vi "Autonomous.vi"() -> ()   [LabVIEW 2016]
doc: "This VI starts when autonomous period begins, and will automatically be terminated when it ends. You can carry out timed or sensor driven operations directly to I/O or to subsystems without needing to return to the caller."
uses:
  <vilib>/Rock Robotics/WPI/ThirdParty/CanMotor/TalonSRX/WPI_CANTalonSRX_BrakeOverride.ctl
  <vilib>/Rock Robotics/WPI/Utilities/WPI_GetSetVariantRefNum.vi
  <vilib>/Rock Robotics/Network Tables/NT Read String.vi
  <vilib>/Rock Robotics/Network Tables/NT Read Number.vi
  Winch/Implementation/Winch Globals.vi
  <vilib>/Rock Robotics/Network Tables/NT Read Boolean.vi
panel:
  in  "stop 3":bool
  in  "stop 2":bool
  out "x-y":u32
  in  "stop":bool
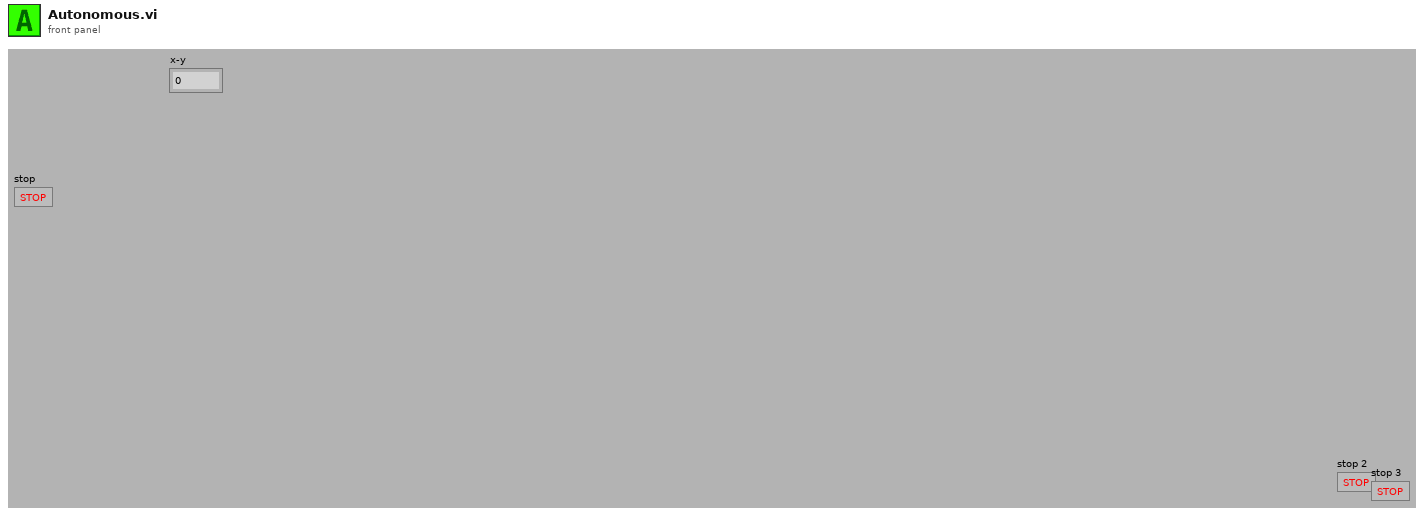
[diagram p1: front panel]
types:
  T1 = typedef "WPI_JoystickDevRef.ctl" = cluster{"Device":T2}
  T2 = typedef "WPI_JoystickDeviceEnum.ctl" = enum16{"USB 0", "USB 1", "USB 2", "USB 3", "USB 4", "USB 5"}
  T3 = typedef "WPI_CANTalonSRX_BrakeOverride.ctl" = enum8{"No Override", "Override to Coast", "Override to Brake"}
  T4 = typedef "WPI_RobotDriveDevRef.ctl" = cluster{"DevStatus":errorcluster, "Motors[]":T5[], "Square Inputs":bool, "Max Output":dbl}
  T5 = typedef "WPI_MotorControlDeviceRef.ctl" = cluster{"DeviceStatus":errorcluster, "Type":T6, "PWM":cluster{"PWM Channel":T7, "DeadBand":T8}, "CAN":cluster{"Device Number":u8, "SetOutput VI Ref":variant, "GetOutput VI Ref":variant, "Enable VI Ref":variant, "Disable VI Ref":variant, "Data":variant}, "Invert":bool}
  T6 = typedef "WPI_MotorControlType.ctl" = enum16{"PWM", "CAN"}
  T7 = typedef "FPGA_DIOPWMChannel.ctl" = enum8{"PWM 0", "PWM 1", "PWM 2", "PWM 3", "PWM 4", "PWM 5", "PWM 6", "PWM 7", "PWM 8", "PWM 9", "PWM MXP 0", "PWM MXP 1", "PWM MXP 2", "PWM MXP 3", "PWM MXP 4", "PWM MXP 5", "PWM MXP 6", "PWM MXP 7", "PWM MXP 8", "PWM MXP 9", "Invalid"}
  T8 = typedef "WPI_PWMDeadband.ctl" = cluster{"Name":string, "maxPositivePwm":i32, "minPositivePwm":i32, "centerPwm":i32, "maxNegativePwm":i32, "minNegativePwm":i32, "angularRange":u16}
  T9 = typedef "WPI_ServoDeviceRef.ctl" = cluster{"DeviceStatus":errorcluster, "PWM Channel":T7, "DeadBand":T8}
  T10 = typedef "Command Status Info.ctl" = cluster{"Name":string, "Status":T11, "notifier out":T12}
  T11 = typedef "Completion Status.ctl" = enum16{"Successful", "Aborted", "Incomplete"}
  T12 = typedef "Completion Notifier.ctl" = refnum<notifier>
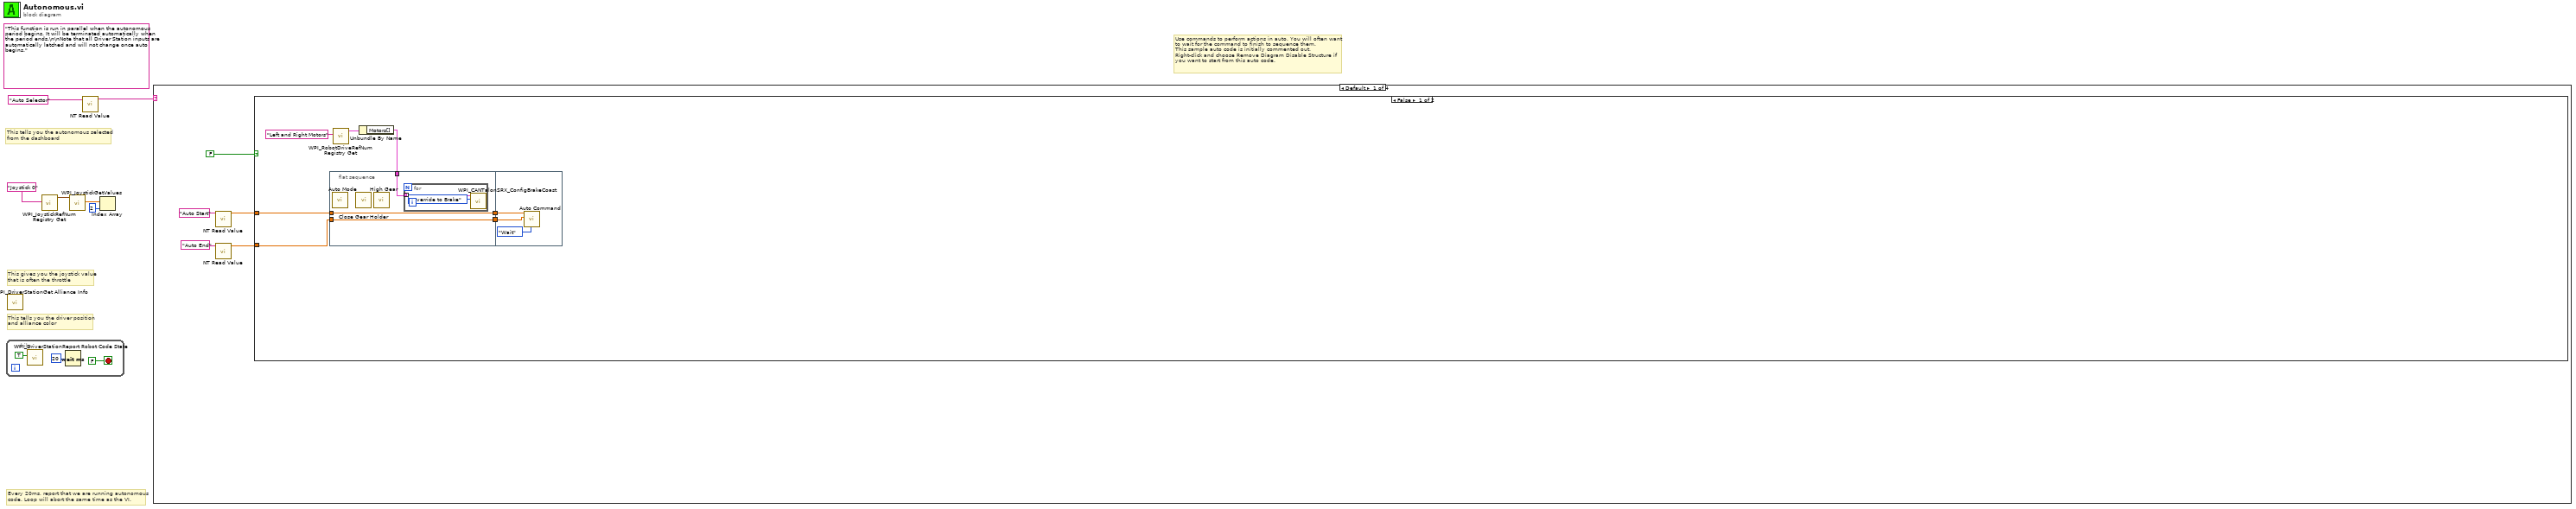
[diagram p0: block diagram]
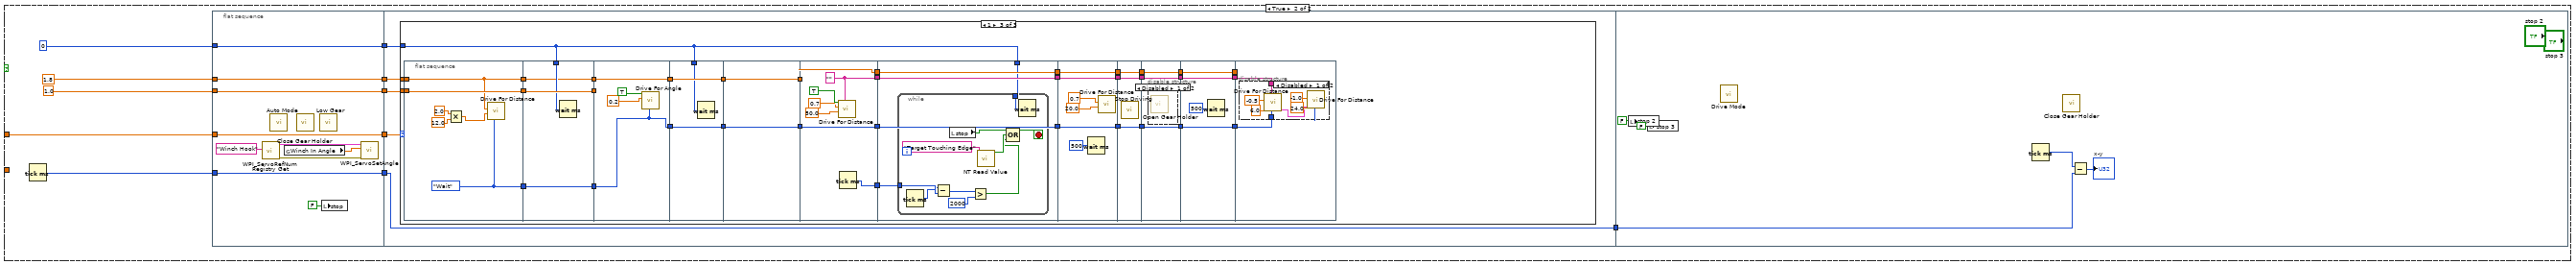
[diagram p2: hidden frame]
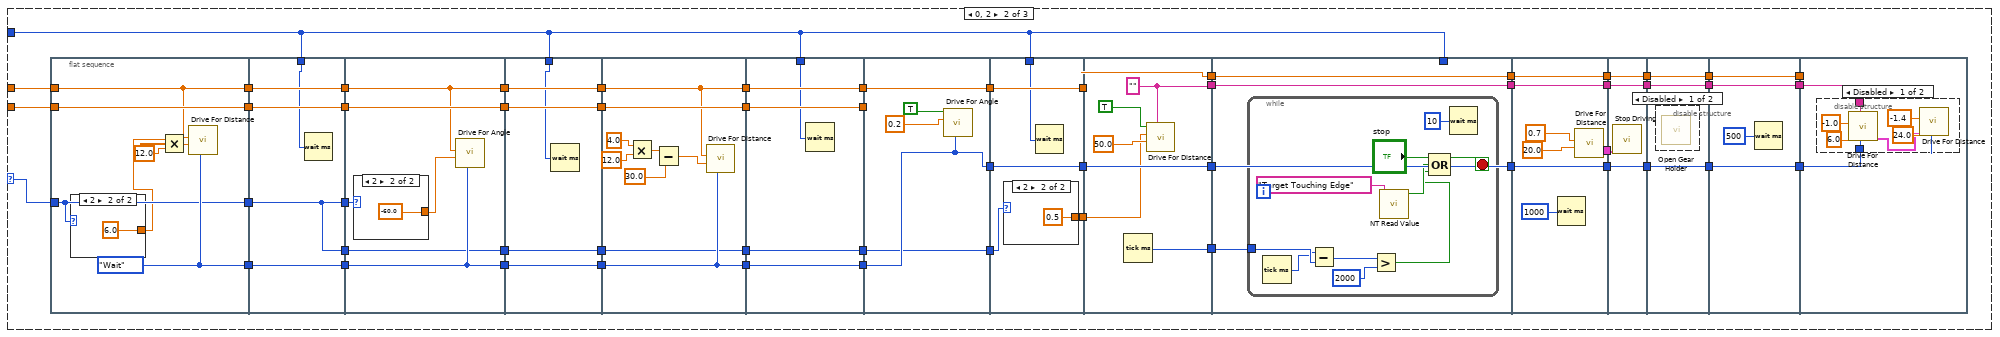
[diagram p4: hidden frame]
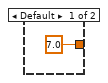
[diagram p5: hidden frame]
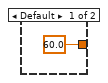
[diagram p6: hidden frame]
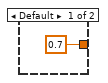
[diagram p7: hidden frame]
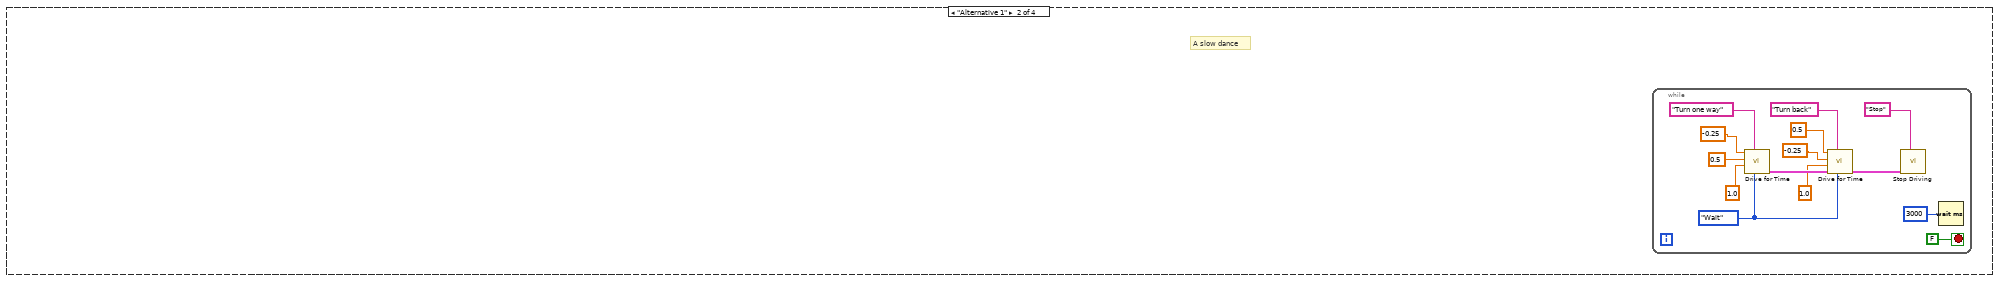
[diagram p12: hidden frame]
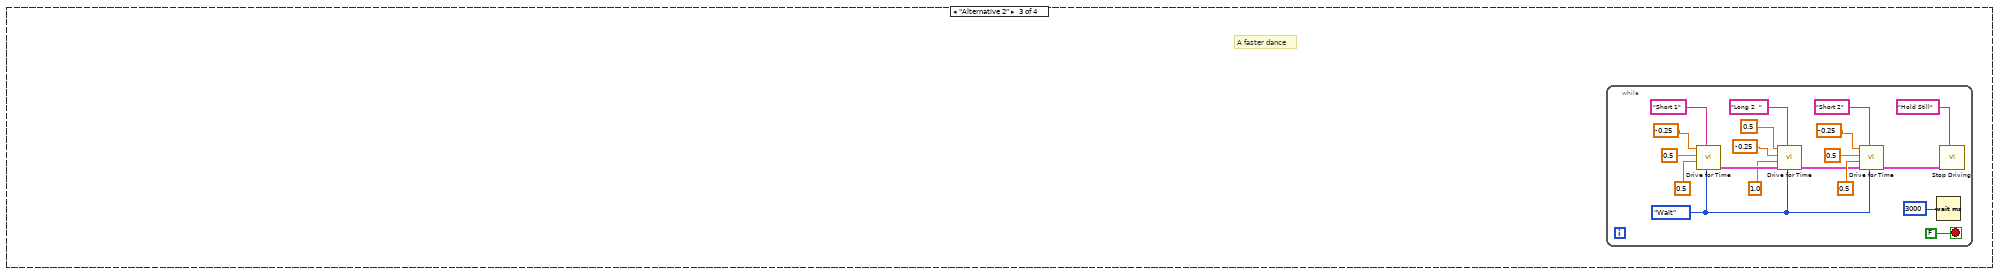
[diagram p13: hidden frame]
diagram:
  (unwired) "This function is run in parallel when the autonomous period begins. It will be terminated automatically when the period ends.\n\nNote that all Driver Station inputs are automatically latched and will not change once auto begins."
  # "This tells you the autonomous selected\nfrom the dashboard"
  # "Every 20ms, report that we are running autonomous\ncode. Loop will abort the same time as the VI."
  # "This gives you the joystick value\nthat is often the throttle"
  # "Use commands to perform actions in auto. You will often want\nto wait for the command to finish to sequence them.\nThis sample auto code is initially commented out. \nRight-click and choose Remove Diagram Disable Structure if\nyou want to start from this auto code."
  # "This tells you the driver position\nand alliance color"
  n1 = while {
    stop <- FALSE stop-if-true
    n2 = call <vilib>:"WPI_DriverStationReport Robot Code State.vi"("Autonomous"=TRUE) -> ()  [unwired: 10 in, 1 out]
    n3 = Wait (ms)(milliseconds to wait=u32 20) -> ()  [unwired: 1 out]
  }
  n4 = call <vilib>:"WPI_DriverStationGet Alliance Info.vi"() -> ()  [unwired: 12 out]
  n5 = call <vilib>:"WPI_JoystickRefNum Registry Get.vi"("refnum name"="Joystick 0") -> ("JoystickDevRef"=w5:T1)  [unwired: 1 in, 9 out]
  n6 = call <vilib>:"WPI_JoystickGetValues.vi"("JoystickDevRef"=w5) -> ("Axes"=w4:dbl[])  [unwired: 6 in, 4 out]
  n7 = call-poly <vilib>:"NT Read Value.vi"("Name"="Auto Selector") -> ("String"=w1:string)  [unwired: 9 in, 1 out]
  n8 = Index Array(array=w4, index=2) -> ()  [unwired: 1 out]
  n9 = case shown="Default" w1 {
    frame Default {
      n10 = call-poly <vilib>:"NT Read Value.vi"("Name"="Auto Start") -> ("Numeric"=w12:dbl)  [unwired: 9 in, 1 out]
      n11 = call-poly <vilib>:"NT Read Value.vi"("Name"="Auto End") -> ("Numeric"=w10:dbl)  [unwired: 9 in, 1 out]
      n12 = case shown="False" FALSE {
        tunnel: w12 -> [w21 w30]
        tunnel: w10 -> [w18 _]
        frame False {
          n13 = flat-sequence {
            tunnel: w21 -> [w24]
            tunnel: [w24] -> w20
            tunnel: w18 -> [w23]
            tunnel: [w23] -> w19
            tunnel: w15 -> [w22]
            tunnel: w20 -> [w29]
            tunnel: w19 -> [w27]
            frame #0 {
              n14 = call "Auto Mode.vi"() -> ()  [unwired: 12 in]
              n15 = call "Close Gear Holder.vi"() -> ()  [unwired: 12 in]
              n16 = call "High Gear.vi"() -> ()  [unwired: 12 in]
              n17 = for {
                tunnel: w22 -> [w25] mode=indexing
                n18 = call <vilib>:"WPI_CANTalonSRX_ConfigBrakeCoast.vi"("Brake / Coast Mode"=WPI_CANTalonSRX_BrakeOverride."Override to Brake", "CAN Talon SRX Ref"=w25) -> ()  [unwired: 8 in, 2 out]
              }
            }
            frame #1 {
              n19 = call "Auto Command.vi"("Synchronization"=enum16{"Start", "Wait"}."Wait", "End Position"=w27, "Start Position"=w29) -> ()  [unwired: 7 in, 2 out]
            }
          }
          n20 = call <vilib>:"WPI_RobotDriveRefNum Registry Get.vi"("refnum name"="Left and Right Motors") -> ("RobotDriveDevRef"=w16:T4)  [unwired: 9 in, 1 out]
          n21 = Unbundle By Name(w16) -> ("Motors[]"=w15:T5[])
        }
        frame True {
          n22 = Tick Count (ms)() -> (millisecond timer value=w31:u32)
          n23 = flat-sequence {
            tunnel: w31 -> [w47]
            tunnel: u32 0 ("milliseconds to wait") -> [w48]
            tunnel: 1.0 ("Speed") -> [w49]
            tunnel: 1.8 ("Speed") -> [w50]
            tunnel: [w50] -> w40
            tunnel: [w49] -> w39
            tunnel: [w48] -> w38
            tunnel: [w47] -> w37
            tunnel: [w42] -> w36
            tunnel: w30 -> [w42]
            tunnel: w40 -> [w55]
            tunnel: w39 -> [w54]
            tunnel: w38 -> [w53]
            tunnel: w37 -> [w52]
            tunnel: [w52] -> w35
            tunnel: w36 -> [w51]
            tunnel: w35 -> [w314]
            frame #0 {
              n24 = call <vilib>:"WPI_ServoRefNum Registry Get.vi"("refnum name"="Winch Hook") -> ("error out"=w46:errorcluster, "ServoDeviceRef"=w45:T9)  [unwired: 9 in]
              n25 = call "Auto Mode.vi"() -> ()  [unwired: 12 in]
              n26 = global read "Winch Globals.vi" "Winch In Angle"() -> (w43:dbl)
              n27 = call "Close Gear Holder.vi"() -> ()  [unwired: 12 in]
              n28 = call "Low Gear.vi"() -> ()  [unwired: 12 in]
              n29 = local write "stop"(FALSE ("stop")) -> ()
              n30 = call <vilib>:"WPI_ServoSetAngle.vi"("error in (no error)"=w46, "Angle"=w43, "ServoDeviceRef"=w45) -> ()  [unwired: 7 in, 2 out]
            }
            frame #1 {
              n31 = case shown="1" w51 {
                selector: w51 -> [_ w67 _]
                tunnel: w55 -> [_ w73 w222]
                tunnel: w54 -> [_ w72 w221]
                tunnel: w53 -> [_ w71 w220]
                frame Default {
                }
                frame 0, 2 {
                  n32 = flat-sequence {
                    tunnel: [w115] -> w110
                    tunnel: [w116] -> w109
                    tunnel: [w114] -> w108
                    tunnel: w73 -> [w115]
                    tunnel: w72 -> [w116]
                    tunnel: w67 -> [w112]
                    tunnel: [w112] -> w66
                    tunnel: [w124] -> w107
                    tunnel: [w123] -> w106
                    tunnel: w110 -> [w124]
                    tunnel: w109 -> [w123]
                    tunnel: [w122] -> w105
                    tunnel: w108 -> [w122]
                    tunnel: w71 -> [w121]
                    tunnel: w66 -> [w120]
                    tunnel: [w120] -> w65
                    tunnel: [w120] -> w57
                    tunnel: [w125] -> w104
                    tunnel: [w126] -> w103
                    tunnel: w107 -> [w125]
                    tunnel: w106 -> [w126]
                    tunnel: w105 -> [w130]
                    tunnel: [w130] -> w102
                    tunnel: w65 -> [w128]
                    tunnel: [w127] -> w58
                    tunnel: w57 -> [w127]
                    tunnel: [w137] -> w101
                    tunnel: w104 -> [w137]
                    tunnel: w103 -> [w136]
                    tunnel: [w136] -> w100
                    tunnel: [w135] -> w99
                    tunnel: w102 -> [w135]
                    tunnel: w71 -> [w134]
                    tunnel: [w133] -> w59
                    tunnel: w58 -> [w133]
                    tunnel: w101 -> [w139]
                    tunnel: [w139] -> w70
                    tunnel: w100 -> [w146]
                    tunnel: [w146] -> w69
                    tunnel: w99 -> [w140]
                    tunnel: [w140] -> w68
                    tunnel: [w138] -> w60
                    tunnel: w59 -> [w138]
                    tunnel: w70 -> [w151]
                    tunnel: [w151] -> w98
                    tunnel: w69 -> [w150]
                    tunnel: [w150] -> w97
                    tunnel: w68 -> [w149]
                    tunnel: [w149] -> w96
                    tunnel: w71 -> [w148]
                    tunnel: [w147] -> w61
                    tunnel: w60 -> [w147]
                    tunnel: [w155] -> w95
                    tunnel: [w156] -> w94
                    tunnel: w98 -> [w156]
                    tunnel: w97 -> [_]
                    tunnel: w96 -> [w155]
                    tunnel: [w152] -> w62
                    tunnel: w61 -> [w152]
                    tunnel: w95 -> [w161]
                    tunnel: [w161] -> w93
                    tunnel: [w160] -> w92
                    tunnel: w94 -> [w160]
                    tunnel: w71 -> [w159]
                    tunnel: w62 -> [w158]
                    tunnel: [w157] -> w56
                    tunnel: w93 -> [w169]
                    tunnel: [w169] -> w91
                    tunnel: [w170] -> w90
                    tunnel: w92 -> [w167]
                    tunnel: [w167] -> w89
                    tunnel: [w165] -> w64
                    tunnel: w56 -> [w164]
                    tunnel: w91 -> [w174]
                    tunnel: [w174] -> w88
                    tunnel: w90 -> [w173]
                    tunnel: [w173] -> w87
                    tunnel: w71 -> [_]
                    tunnel: [w172] -> w86
                    tunnel: w89 -> [w172]
                    tunnel: w64 -> [w171]
                    tunnel: w88 -> [w191]
                    tunnel: [w191] -> w85
                    tunnel: w87 -> [w190]
                    tunnel: [w190] -> w84
                    tunnel: [w189] -> w83
                    tunnel: w86 -> [w189]
                    tunnel: [w186] -> w63
                    tunnel: w85 -> [w195]
                    tunnel: [w195] -> w82
                    tunnel: w84 -> [w194]
                    tunnel: [w194] -> w81
                    tunnel: [w193] -> w80
                    tunnel: w83 -> [w193]
                    tunnel: w63 -> [w192]
                    tunnel: w82 -> [w198]
                    tunnel: [w198] -> w79
                    tunnel: w81 -> [w197]
                    tunnel: [w197] -> w78
                    tunnel: [w196] -> w77
                    tunnel: w80 -> [w196]
                    tunnel: w79 -> [w202]
                    tunnel: [w202] -> w76
                    tunnel: w78 -> [w201]
                    tunnel: [w201] -> w75
                    tunnel: [w199] -> w74
                    tunnel: w77 -> [w199]
                    tunnel: w76 -> [w203]
                    tunnel: w75 -> [w204]
                    tunnel: w74 -> [_]
                    frame #0 {
                      w114 = enum16{"Start", "Wait"}."Wait" ("Synchronization")
                      n33 = case shown="2" w112 {
                        tunnel: [7.0 ("Distance") 6.0 ("Distance")] -> w111
                        frame Default {
                        }
                        frame 2 {
                        }
                      }
                      n34 = Multiply(x=w111, y=12.0) -> (x*y=w113:dbl)
                      n35 = call "Drive For Distance.vi"("Synchronization"=w114, "Distance"=w113, "Speed"=w115) -> ()  [unwired: 7 in, 2 out]
                    }
                    frame #1 {
                      n36 = Wait (ms)(milliseconds to wait=w121) -> ()  [unwired: 1 out]
                    }
                    frame #2 {
                      n37 = case shown="2" w128 {
                        tunnel: [60.0 ("Distance") -60.0 ("Distance")] -> w129
                        frame Default {
                        }
                        frame 2 {
                        }
                      }
                      n38 = call "Drive For Angle.vi"("Synchronization"=w130, "Angle"=w129, "Speed"=w125) -> ()  [unwired: 7 in, 2 out]
                    }
                    frame #3 {
                      n39 = Wait (ms)(milliseconds to wait=w134) -> ()  [unwired: 1 out]
                    }
                    frame #4 {
                      n40 = Multiply(x=4.0, y=12.0) -> (x*y=w143:dbl)
                      n41 = Subtract(x=w143, y=30.0) -> (x-y=w145:dbl)
                      n42 = call "Drive For Distance.vi"("Synchronization"=w140, "Distance"=w145, "Speed"=w139) -> ()  [unwired: 7 in, 2 out]
                    }
                    frame #5 {
                      n43 = Wait (ms)(milliseconds to wait=w148) -> ()  [unwired: 1 out]
                    }
                    frame #6 {
                      n44 = call "Drive For Angle.vi"("Synchronization"=w155, "Speed"=0.2 ("x"), "Vision"=TRUE) -> ()  [unwired: 7 in, 2 out]
                    }
                    frame #7 {
                      n45 = case shown="2" w158 {
                        tunnel: [0.7 ("Distance") 0.5 ("Distance")] -> w157
                        frame Default {
                        }
                        frame 2 {
                        }
                      }
                      n46 = Wait (ms)(milliseconds to wait=w159) -> ()  [unwired: 1 out]
                    }
                    frame #8 {
                      w170 = "" ("Description")
                      n47 = Tick Count (ms)() -> (millisecond timer value=w165:u32)
                      n48 = call "Drive For Distance.vi"("Description"=w170, "Distance"=50.0, "Speed"=w164, "Vision"=TRUE) -> ()  [unwired: 6 in, 2 out]
                    }
                    frame #9 {
                      n49 = while {
                        tunnel: w171 -> [w180]
                        stop <- w182 stop-if-true
                        n50 = Tick Count (ms)() -> (millisecond timer value=w179:u32)
                        n51 = Subtract(x=w179, y=w180) -> (x-y=w178:u32)
                        n52 = Greater?(x=w178, y=u32 2000) -> (0:w176:bool)
                        n53 = call-poly <vilib>:"NT Read Value.vi"("Name"="Target Touching Edge") -> ("Boolean"=w181:bool)  [unwired: 9 in, 1 out]
                        n54 = Compound Arithmetic op=OR("stop", w181, w176) -> (w182:bool)
                        n55 = Wait (ms)(milliseconds to wait=u32 10) -> ()  [unwired: 1 out]
                      }
                    }
                    frame #10 {
                      n56 = Wait (ms)(milliseconds to wait=u32 1000) -> ()  [unwired: 1 out]
                      n57 = call "Drive For Distance.vi"("Distance"=20.0, "Speed"=0.7 ("x")) -> ("Command Info Out"=w186:T10)  [unwired: 8 in, 1 out]
                    }
                    frame #11 {
                      n58 = call "Stop Driving.vi"("Command Info In"=w192) -> ()  [unwired: 10 in, 1 out]
                    }
                    frame #12 {
                      n59 = disable-structure shown="Disabled" {
                        frame Disabled {
                          n60 = call "Open Gear Holder.vi"() -> ()  [unwired: 12 in]
                        }
                        frame Enabled {
                        }
                      }
                    }
                    frame #13 {
                      n61 = Wait (ms)(milliseconds to wait=u32 500) -> ()  [unwired: 1 out]
                    }
                    frame #14 {
                      n62 = disable-structure shown="Disabled" {
                        disable-tunnel: w204 -> [w210 _]
                        disable-tunnel: w203 -> [w207 _]
                        frame Disabled {
                          n63 = call "Drive For Distance.vi"("Synchronization"=w207, "Description"=w210, "Distance"=6.0, "Speed"=-1.0) -> ("Command Info Out"=w206:T10)  [unwired: 6 in, 1 out]
                          n64 = call "Drive For Distance.vi"("Synchronization"=w207, "Command Info In"=w206, "Distance"=24.0, "Speed"=-1.4) -> ()  [unwired: 6 in, 2 out]
                        }
                        frame Enabled {
                        }
                      }
                    }
                  }
                }
                frame 1 {
                  n65 = flat-sequence {
                    tunnel: [w251] -> w219
                    tunnel: w222 -> [w250]
                    tunnel: w221 -> [w251]
                    tunnel: [w250] -> w218
                    tunnel: [w249] -> w217
                    tunnel: [w253] -> w245
                    tunnel: w219 -> [w255]
                    tunnel: [w255] -> w244
                    tunnel: [w252] -> w243
                    tunnel: w220 -> [w254]
                    tunnel: w218 -> [w253]
                    tunnel: w217 -> [w252]
                    tunnel: [w257] -> w242
                    tunnel: [w259] -> w241
                    tunnel: w245 -> [w259]
                    tunnel: w244 -> [_]
                    tunnel: w243 -> [w257]
                    tunnel: w242 -> [w262]
                    tunnel: [w262] -> w216
                    tunnel: [w261] -> w214
                    tunnel: w241 -> [w261]
                    tunnel: w220 -> [w260]
                    tunnel: w216 -> [w263]
                    tunnel: [w263] -> w215
                    tunnel: w214 -> [w264]
                    tunnel: [w264] -> w213
                    tunnel: w215 -> [w270]
                    tunnel: [w270] -> w240
                    tunnel: [w271] -> w239
                    tunnel: w213 -> [w267]
                    tunnel: [w267] -> w238
                    tunnel: [w265] -> w212
                    tunnel: w240 -> [w276]
                    tunnel: [w276] -> w237
                    tunnel: w239 -> [w275]
                    tunnel: [w275] -> w236
                    tunnel: w220 -> [w273]
                    tunnel: [w274] -> w235
                    tunnel: w238 -> [w274]
                    tunnel: w212 -> [w272]
                    tunnel: w237 -> [w292]
                    tunnel: [w292] -> w234
                    tunnel: w236 -> [w291]
                    tunnel: [w291] -> w233
                    tunnel: [w290] -> w232
                    tunnel: w235 -> [w290]
                    tunnel: w234 -> [w295]
                    tunnel: [w295] -> w231
                    tunnel: w233 -> [w294]
                    tunnel: [w294] -> w230
                    tunnel: [w293] -> w229
                    tunnel: w232 -> [w293]
                    tunnel: w231 -> [w298]
                    tunnel: [w298] -> w228
                    tunnel: w230 -> [w297]
                    tunnel: [w297] -> w227
                    tunnel: [w296] -> w226
                    tunnel: w229 -> [w296]
                    tunnel: w228 -> [w302]
                    tunnel: [w302] -> w225
                    tunnel: w227 -> [w301]
                    tunnel: [w301] -> w224
                    tunnel: [w299] -> w223
                    tunnel: w226 -> [w299]
                    tunnel: w225 -> [w303]
                    tunnel: w224 -> [w304]
                    tunnel: w223 -> [_]
                    frame #0 {
                      w249 = enum16{"Start", "Wait"}."Wait" ("Synchronization")
                      n66 = Multiply(x=2.0, y=12.0) -> (x*y=w246:dbl)
                      n67 = call "Drive For Distance.vi"("Synchronization"=w249, "Distance"=w246, "Speed"=w250) -> ()  [unwired: 7 in, 2 out]
                    }
                    frame #1 {
                      n68 = Wait (ms)(milliseconds to wait=w254) -> ()  [unwired: 1 out]
                    }
                    frame #2 {
                      n69 = call "Drive For Angle.vi"("Synchronization"=w257, "Speed"=0.2 ("x"), "Vision"=TRUE) -> ()  [unwired: 7 in, 2 out]
                    }
                    frame #3 {
                      n70 = Wait (ms)(milliseconds to wait=w260) -> ()  [unwired: 1 out]
                    }
                    frame #4 {
                    }
                    frame #5 {
                      w271 = "" ("Description")
                      n71 = call "Drive For Distance.vi"("Description"=w271, "Distance"=50.0, "Speed"=0.7 ("x"), "Vision"=TRUE) -> ()  [unwired: 6 in, 2 out]
                      n72 = Tick Count (ms)() -> (millisecond timer value=w265:u32)
                    }
                    frame #6 {
                      n73 = while {
                        tunnel: w273 -> [w283]
                        tunnel: w272 -> [w282]
                        stop <- w285 stop-if-true
                        n74 = Tick Count (ms)() -> (millisecond timer value=w281:u32)
                        n75 = Subtract(x=w281, y=w282) -> (x-y=w280:u32)
                        n76 = local read "stop"() -> (w277:bool)
                        n77 = Greater?(x=w280, y=u32 2000) -> (0:w278:bool)
                        n78 = call-poly <vilib>:"NT Read Value.vi"("Name"="Target Touching Edge") -> ("Boolean"=w284:bool)  [unwired: 9 in, 1 out]
                        n79 = Compound Arithmetic op=OR(w277, w284, w278) -> (w285:bool)
                        n80 = Wait (ms)(milliseconds to wait=w283) -> ()  [unwired: 1 out]
                      }
                    }
                    frame #7 {
                      n81 = Wait (ms)(milliseconds to wait=u32 500) -> ()  [unwired: 1 out]
                      n82 = call "Drive For Distance.vi"("Distance"=20.0, "Speed"=0.7 ("x")) -> ()  [unwired: 8 in, 2 out]
                    }
                    frame #8 {
                      n83 = call "Stop Driving.vi"() -> ()  [unwired: 11 in, 1 out]
                    }
                    frame #9 {
                      n84 = disable-structure shown="Disabled" {
                        frame Disabled {
                          n85 = call "Open Gear Holder.vi"() -> ()  [unwired: 12 in]
                        }
                        frame Enabled {
                        }
                      }
                    }
                    frame #10 {
                      n86 = Wait (ms)(milliseconds to wait=u32 500) -> ()  [unwired: 1 out]
                    }
                    frame #11 {
                      n87 = disable-structure shown="Disabled" {
                        disable-tunnel: w304 -> [w310 _]
                        disable-tunnel: w303 -> [w307 _]
                        frame Disabled {
                          n88 = call "Drive For Distance.vi"("Synchronization"=w307, "Description"=w310, "Distance"=6.0, "Speed"=-0.5) -> ("Command Info Out"=w306:T10)  [unwired: 6 in, 1 out]
                          n89 = call "Drive For Distance.vi"("Synchronization"=w307, "Command Info In"=w306, "Distance"=24.0, "Speed"=-1.0) -> ()  [unwired: 6 in, 2 out]
                        }
                        frame Enabled {
                        }
                      }
                    }
                  }
                }
              }
            }
            frame #2 {
              n90 = local write "stop 2"(FALSE ("stop")) -> ()
              n91 = local write "stop 3"(FALSE ("stop")) -> ()
              n92 = call "Drive Mode.vi"() -> ()  [unwired: 12 in]
              n93 = Tick Count (ms)() -> (millisecond timer value=w315:u32)
              n94 = call "Close Gear Holder.vi"() -> ()  [unwired: 12 in]
              n95 = Subtract(x=w315, y=w314) -> (x-y=→"x-y":u32)
            }
          }
        }
      }
    }
    frame "Alternative 1" {
      # "A slow dance"
      n96 = while {
        stop <- FALSE stop-if-true
        w321 = enum16{"Start", "Wait"}."Wait" ("Synchronication")
        n97 = call "Drive for Time.vi"("Synchronization"=w321, "Description"="Turn one way", "Seconds"=1.0 ("Delay (s)"), "Right Speed"=0.5 ("X axis value"), "Left Speed"=-0.25 ("X axis value")) -> ("Command Info Out"=w330:T10)  [unwired: 5 in, 1 out]
        n98 = call "Drive for Time.vi"("Synchronization"=w321, "Description"="Turn back", "Command Info In"=w330, "Seconds"=1.0 ("Delay (s)"), "Right Speed"=-0.25 ("X axis value"), "Left Speed"=0.5 ("X axis value")) -> ("Command Info Out"=w320:T10)  [unwired: 4 in, 1 out]
        n99 = call "Stop Driving.vi"("Description"="Stop", "Command Info In"=w320) -> ()  [unwired: 9 in, 1 out]
        n100 = Wait (ms)(milliseconds to wait=u32 3000 ("millisecond timer value")) -> ()  [unwired: 1 out]
      }
    }
    frame "Alternative 2" {
      # "A faster dance"
      n101 = while {
        stop <- FALSE stop-if-true
        w331 = enum16{"Start", "Wait"}."Wait" ("Synchronication")
        n102 = call "Drive for Time.vi"("Synchronization"=w331, "Description"="Short 1", "Seconds"=0.5 ("Delay (s)"), "Right Speed"=0.5 ("X axis value"), "Left Speed"=-0.25 ("X axis value")) -> ("Command Info Out"=w349:T10)  [unwired: 5 in, 1 out]
        n103 = call "Drive for Time.vi"("Synchronization"=w331, "Description"="Long 2  ", "Command Info In"=w349, "Seconds"=1.0 ("Delay (s)"), "Right Speed"=-0.25 ("X axis value"), "Left Speed"=0.5 ("X axis value")) -> ("Command Info Out"=w333:T10)  [unwired: 4 in, 1 out]
        n104 = call "Drive for Time.vi"("Synchronization"=w331, "Description"="Short 2", "Command Info In"=w333, "Seconds"=0.5 ("Delay (s)"), "Right Speed"=0.5 ("X axis value"), "Left Speed"=-0.25 ("X axis value")) -> ("Command Info Out"=w332:T10)  [unwired: 4 in, 1 out]
        n105 = Wait (ms)(milliseconds to wait=u32 3000 ("millisecond timer value")) -> ()  [unwired: 1 out]
        n106 = call "Stop Driving.vi"("Description"="Hold Still", "Command Info In"=w332) -> ()  [unwired: 9 in, 1 out]
      }
    }
    frame "Your Turn" {
    }
  }
